vi "Load Program Process AHU.vi"(0 "Enable":bool=TRUE, 7 "error in (no error)":errorcluster) -> (1 "Speed Command Test":bool, 3 "Enable Test":bool, 4 "Temperature Control Algorithm Test":bool, 5 "Burn-in Test":bool, 8 "Auxiliary":bool, 9 "Temperature Sensor Calibration Test":bool, 12 "Communication Test":bool, 13 "Sealing Test":bool, 14 "CANBus Resistance Test":bool, 15 "Bonding Resistance":bool, 16 "Insulation Resistance Test":bool, 17 "Weight Check":bool, 20 "Power Supply Voltages":bool, 21 "Power Supply Testing":bool, 22 "Stop Time Test":bool, 23 "Manufacturing Defects":bool, 24 "Visual Inspection":bool, 25 "OK":bool, 26 "Automation":bool, 27 "error out":errorcluster)   [LabVIEW 2017]
doc: "Displays a standard dialog box that prompts users to enter information, such as a user name and password.\n--------------------\n\nThis Express VI is configured as follows:\n\nMessage to Display to the User:Please select the test(s) you want to execute(s).\nThe inputs are: \nCheckbox: Visual Inspection\nCheckbox: Manufacturing Defects\nCheckbox: Power Supply Testing\nCheckbox: Power Supply Voltages\nCheckbox: Functional Test Procedure\nCheckbox: Insulation Resistance Test\nCheckbox: Bonding Resistance\nCheckbox: CANBus Resistance Test\nCheckbox: Sealing Test\nCheckbox: Communication Test"
panel:
  in  "Stop Time Test":bool
  in  "Temperature Control Algorithm Test":bool caption="Sealing Test"
  in  "Burn-in Test":bool caption="Communication Test"
  in  "Enable Test":bool caption="Sealing Test"
  in  "Speed Command Test":bool caption="CANBus Resistance Test"
  in  "Temperature Sensor Calibration Test":bool caption="Bonding Resistance"
  in  "Auxiliary":bool
  in  "Communication Test":bool
  in  "Sealing Test":bool
  in  "CANBus Resistance Test":bool
  in  "Bonding Resistance":bool
  in  "Insulation Resistance Test":bool
  in  "Weight Check":bool
  in  "Power Supply Voltages":bool
  in  "Power Supply Testing":bool
  in  "Manufacturing Defects":bool
  in  "Visual Inspection":bool
  out "String":string="Please select the test(s) you want to execute(s)."
  in  "Cancel":bool
  in  "OK2":bool
  in  "Automation":bool caption="OK1"
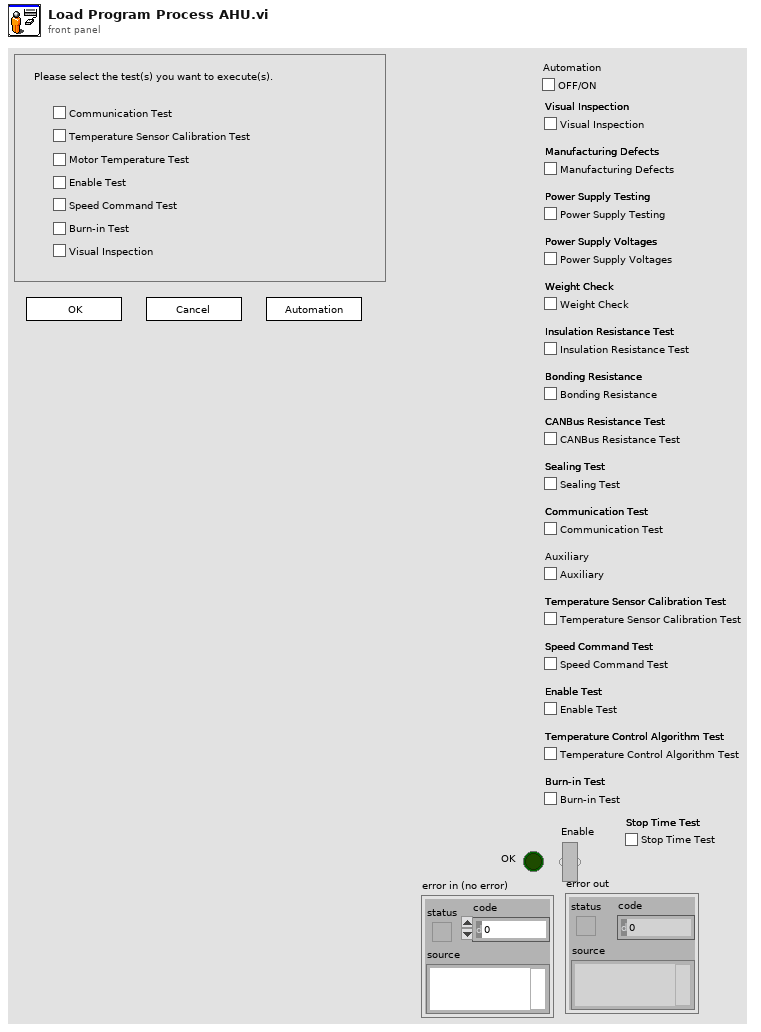
[diagram p1: front panel]
types:
  T1 = cluster{"Input Name":string, "Input Data Type":i32}[]
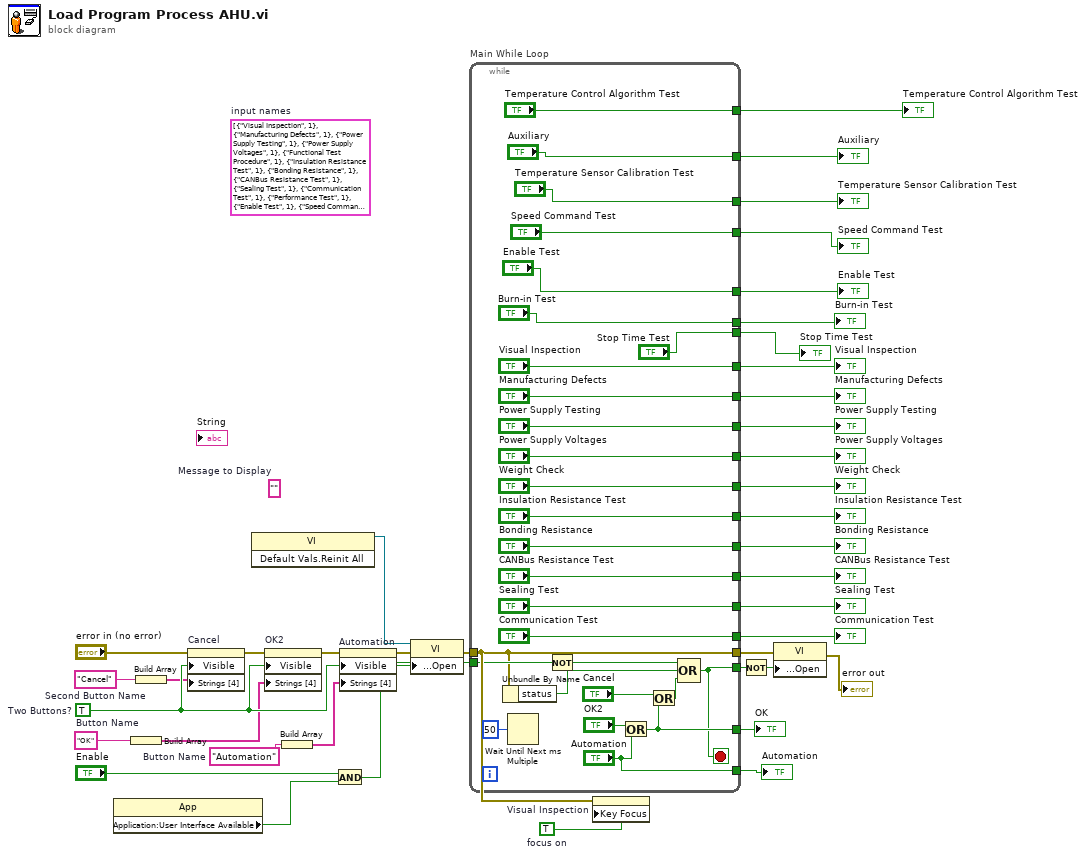
[diagram p0: block diagram]
diagram:
  w5 = "Automation"  # Button Name
  w21 = TRUE  # focus on
  (unwired) T1 [{"Input Name"="Visual Inspection", "Input Data Type"=1}, {"Input Name"="Manufacturing Defects", "Input Data Type"=1}, {"Input Name"="Power Supply Testing", "Input Data Type"=1}, {"Input Name"="Power Supply Voltages", "Input Data Type"=1}, {"Input Name"="Functional Test Procedure", "Input Data Type"=1}, {"Input Name"="Insulation Resistance Test", "Input Data Type"=1}, {"Input Name"="Bonding Resistance", "Input Data Type"=1}, {"Input Name"="CANBus Resistance Test", "Input Data Type"=1}, {"Input Name"="Sealing Test", "Input Data Type"=1}, {"Input Name"="Communication Test", "Input Data Type"=1}, {"Input Name"="Performance Test", "Input Data Type"=1}, {"Input Name"="Enable Test", "Input Data Type"=1}, {"Input Name"="Speed Command Test", "Input Data Type"=1}, {"Input Name"="Temperature Sensor Calibration Test", "Input Data Type"=1}, {"Input Name"="Temperature Control Algorithm Test", "Input Data Type"=1}, {"Input Name"="Burn-in Test ", "Input Data Type"=1}]  # input names
  w33 = "Cancel"  # Second Button Name
  w32 = "OK"  # Button Name
  (unwired) ""  # Message to Display
  w40 = TRUE  # Two Buttons?
  n1 = property class="App"() -> ("Application:User Interface Available"=w24:bool)  [unwired: 2 in, 2 out]
  n2 = Build Array(w32) -> (w7:string[])
  n3 = Build Array(w33) -> (w34:string[])
  n4 = property on="Cancel" class="Bool"(error in="error in (no error)", "Visible"=w40, "Strings [4]"=w34) -> (error out=w38:errorcluster)  [unwired: 1 in, 1 out]
  n5 = invoke class="VI" method="Default Vals.Reinit All"() -> (reference out=w23:refnum<vi>)  [unwired: 3 in, 2 out]
  n6 = property on="OK2" class="Bool"(error in=w38, "Visible"=w40, "Strings [4]"=w7) -> (error out=w37:errorcluster)  [unwired: 1 in, 1 out]
  n7 = Build Array(w5) -> (w6:string[])
  n8 = And(x="Enable", y=w24) -> (x .and. y?=w25:bool)
  n9 = property on="Automation" class="Bool"(error in=w37, "Visible"=w40, "Strings [4]"=w6) -> (error out=w31:errorcluster)  [unwired: 1 in, 1 out]
  n10 = property class="VI"(reference=w23, error in=w31, "Front Panel Window:Open"=w25) -> (error out=w30:errorcluster)  [unwired: 1 out]
  n11 = while "Main While Loop" {
    tunnel: [w65] -> w39
    tunnel: w25 -> [w64]
    tunnel: [w62] -> w35
    tunnel: w30 -> [w61]
    tunnel: [w61] -> w28
    tunnel: ["Visual Inspection"] -> w22
    tunnel: ["Manufacturing Defects"] -> w20
    tunnel: ["Power Supply Testing"] -> w19
    tunnel: ["Power Supply Voltages"] -> w18
    tunnel: ["Weight Check"] -> w17
    tunnel: ["Insulation Resistance Test"] -> w16
    tunnel: ["Bonding Resistance"] -> w15
    tunnel: ["CANBus Resistance Test"] -> w14
    tunnel: ["Sealing Test"] -> w13
    tunnel: ["Communication Test"] -> w12
    tunnel: ["Auxiliary"] -> w11
    tunnel: ["Temperature Sensor Calibration Test"] -> w10
    tunnel: ["Speed Command Test"] -> w9
    tunnel: ["Enable Test"] -> w8
    tunnel: ["Burn-in Test"] -> w2
    tunnel: ["Temperature Control Algorithm Test"] -> w1
    tunnel: ["Automation"] -> w4
    tunnel: ["Stop Time Test"] -> w3
    stop <- w62 stop-if-true
    n12 = Unbundle By Name(w61) -> ("status"=w59:bool)
    n13 = Wait Until Next ms Multiple(millisecond multiple=u32 50) -> ()  [unwired: 1 out]
    n14 = Not(x=w64) -> (.not. x?=w63:bool)
    n15 = Or(x="OK2", y="Automation") -> (x .or. y?=w65:bool)
    n16 = Or(x="Cancel", y=w65) -> (x .or. y?=w60:bool)
    n17 = Compound Arithmetic op=OR(w63, w59, w60) -> (w62:bool)
  }
  "OK" <- w39
  "Visual Inspection" <- w22
  "Manufacturing Defects" <- w20
  "Power Supply Testing" <- w19
  "Power Supply Voltages" <- w18
  "Weight Check" <- w17
  "Insulation Resistance Test" <- w16
  "Bonding Resistance" <- w15
  "CANBus Resistance Test" <- w14
  "Sealing Test" <- w13
  "Communication Test" <- w12
  "Auxiliary" <- w11
  "Temperature Sensor Calibration Test" <- w10
  "Speed Command Test" <- w9
  "Enable Test" <- w8
  "Temperature Control Algorithm Test" <- w1
  "Burn-in Test" <- w2
  "Automation" <- w4
  "Stop Time Test" <- w3
  n18 = property on="Visual Inspection" class="Bool (strict)"(error in=w30, "Key Focus"=w21) -> ()  [unwired: 1 in, 2 out]
  n19 = Not(x=w35) -> (.not. x?=w36:bool)
  n20 = property class="VI"(error in=w28, "Front Panel Window:Open"=w36) -> (error out=→"error out":errorcluster)  [unwired: 1 in, 1 out]
